vi "1-4 난수 플롯(이벤트).vi"() -> ()   [LabVIEW 2014]
doc: "이 템플릿을 사용하여 사용자 인터페이스 이벤트 핸들러 디자인 패턴을 생성합니다. 대화 상자 및 다른 사용자 인터페이스에 대하여 이 패턴을 사용합니다. 또한, VI가 사용자 인터페이스 이벤트를 같은 방법으로 다룰 수 있는, 사용자 정의 이벤트를 생성하고 실행할 수 있습니다."
panel:
  in  "확인":bool caption="정지"
  in  "stop":bool caption="정지"
  out "웨이브폼 차트":dbl(graph)
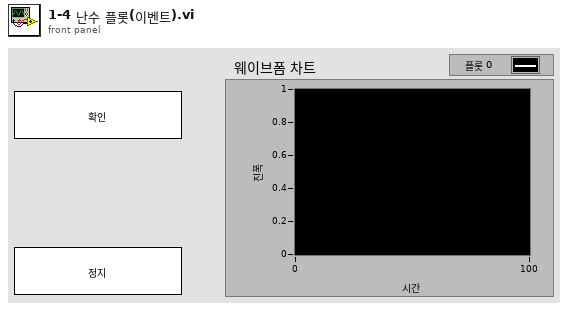
[diagram p1: front panel]
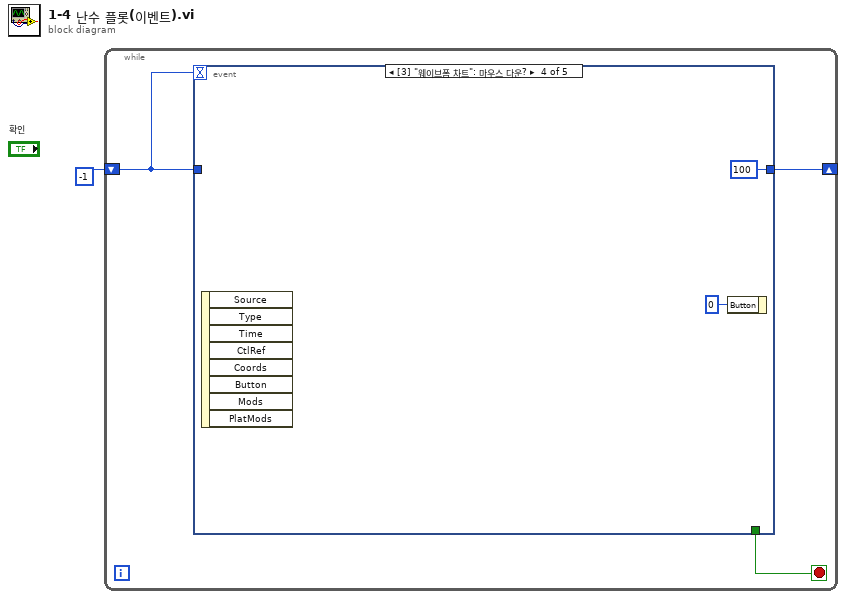
[diagram p0: block diagram]
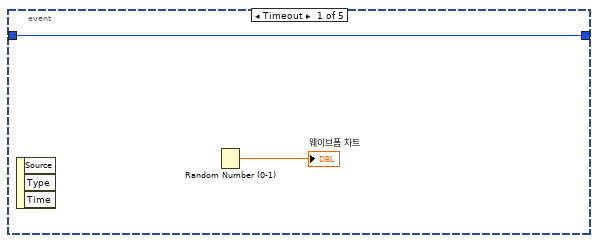
[diagram p2: hidden frame]
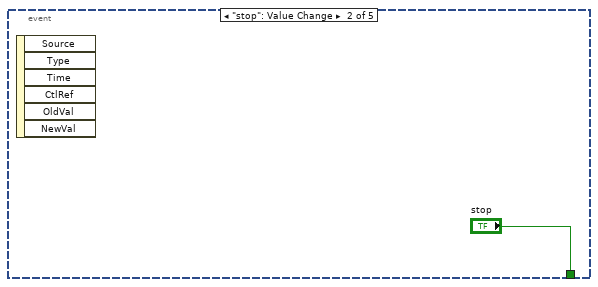
[diagram p3: hidden frame]
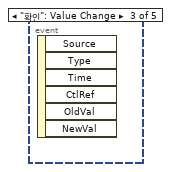
[diagram p4: hidden frame]
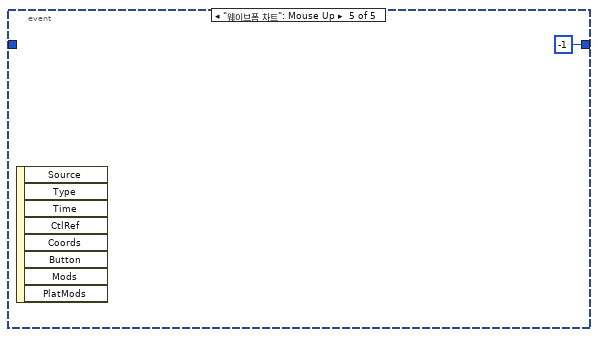
[diagram p5: hidden frame]
diagram:
  n1 = while {
    shift-right: [w3] -> _
    shift-left: -1 -> [w2]
    stop <- w4 stop-if-true
    n2 = event shown="[3] \"웨이브폼 차트\": 마우스 다운?" {
      selector: _ -> [_ _ _ _ _]
      dyn-events: _ -> [_ _ _ _ _]
      timeout: w2 -> [_ _ _ _ _]
      tunnel: [_ "stop" _ _ _] -> w4
      tunnel: [w6 _ _ 100 -1] -> w3
      tunnel: w2 -> [w6 _ _ _ _]
      event Timeout {
        n3 = event-data() -> ()  [unwired: 1 in, 3 out]
        n4 = Random Number (0-1)() -> (number: 0 to 1=→"웨이브폼 차트":dbl)
      }
      event "stop": Value Change {
        n5 = event-data() -> ()  [unwired: 1 in, 6 out]
      }
      event "확인": Value Change {
        n6 = event-data() -> ()  [unwired: 1 in, 6 out]
      }
      event "웨이브폼 차트": Mouse Down? {
        n7 = event-data() -> ()  [unwired: 1 in, 8 out]
        n8 = event-data("Button"=u16 0 ("버튼")) -> ()  [unwired: 1 in, 1 out]
      }
      event "웨이브폼 차트": Mouse Up {
        n9 = event-data() -> ()  [unwired: 1 in, 8 out]
      }
    }
  }
